vi "Fibonacci.vi"(11 "n":dbl) -> (3 "n'th Fibonacci number":dbl)   [LabVIEW 2017]
doc: "VI that generates the n'th Fibonacci number"
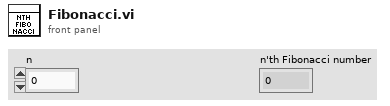
[diagram p1: front panel]
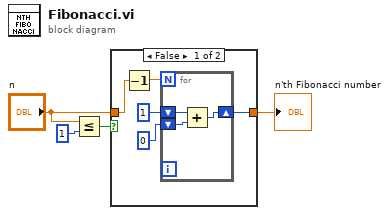
[diagram p0: block diagram]
diagram:
  n1 = Less Or Equal?(x="n", y=1) -> (x <= y?=w2:bool)
  n2 = case shown="False" w2 {
    tunnel: "n" -> [w7 w13]
    tunnel: [w5 w13] -> w1
    frame False {
      n3 = Decrement(x=w7) -> (x-1=w6:dbl)
      n4 = for {
        N: w6 -> [_]
        shift-right: [w10] -> w5
        shift-left: 1 -> [w12]
        shift-left: 0 -> [w11]
        n5 = Add(x=w12, y=w11) -> (x+y=w10:i32)
      }
    }
    frame True {
    }
  }
  "n'th Fibonacci number" <- w1
